vi "Load Harmonics from Test Parameter.vi"(8 "error in (no error)":errorcluster, 11 "Harmonics in":refnum<class "Harmonics.lvclass">) -> (0 "error out":errorcluster, 3 "Harmonics out":refnum<class "Harmonics.lvclass">)   [LabVIEW 2018, in "Harmonics.lvlib" / "Harmonics.lvclass"]
uses:
  Harmonics.lvclass
  C:/Sequence Automation/Plugins/Measurement Interface.lvlibp/Measurement Interface.lvclass
  Harmonics.lvclass/Harmonics.ctl
  Protected Methods/Write Harmonics.vi
  Plugins/Measurement Interface.lvlibp/Private Methods/Measurement Parameters/Read Measurement Parameters.vi
  <vilib>/Analysis/1siggen.llb/Ramp Pattern by Delta.vi
  Plugins/String Database.lvlibp/String Database.lvclass
  <vilib>/Analysis/NI_AALBase.lvlib
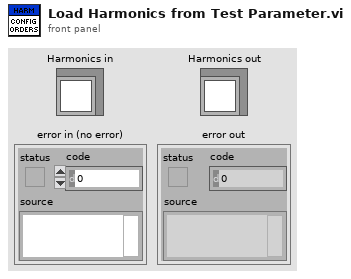
[diagram p1: front panel]
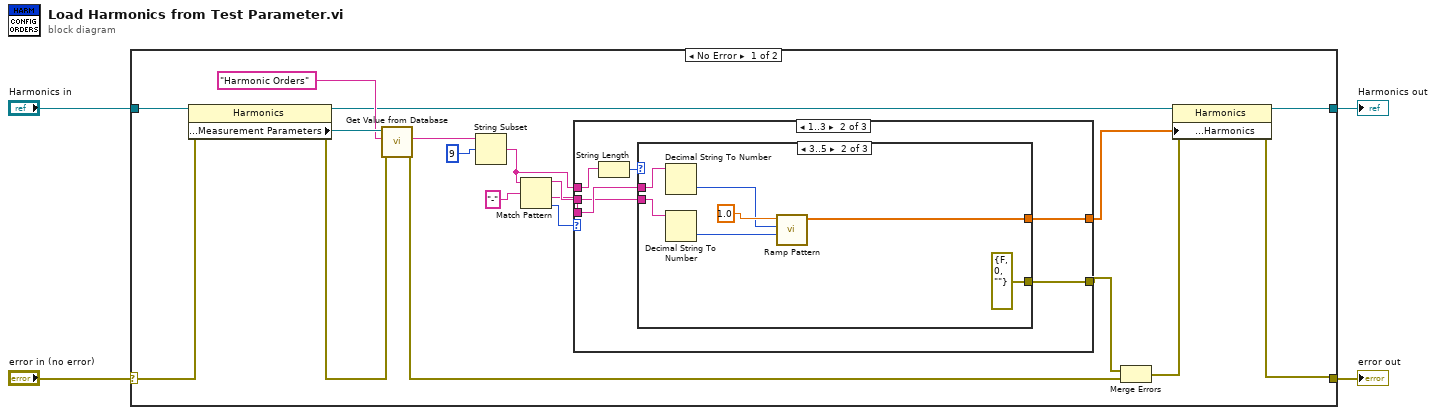
[diagram p0: block diagram]
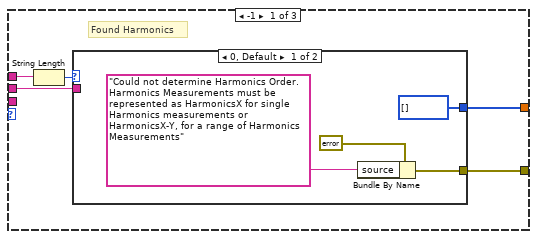
[diagram p2: hidden frame]
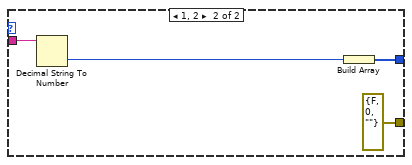
[diagram p3: hidden frame]
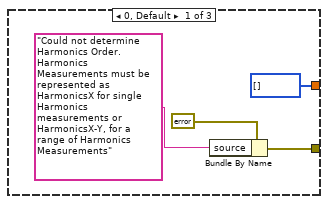
[diagram p4: hidden frame]
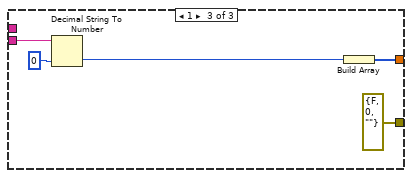
[diagram p5: hidden frame]
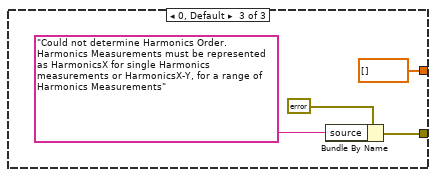
[diagram p6: hidden frame]
diagram:
  n1 = case shown="No Error" "error in (no error)" {
    selector: "error in (no error)" -> [w23 w64]
    tunnel: [w17 w64] -> w3
    tunnel: [w15 w63] -> w1
    tunnel: "Harmonics in" -> [w22 w63]
    frame No Error {
      n2 = property class="Harmonics"(reference=w22, error in=w23) -> (reference out=w16:refnum<class "Harmonics.lvclass">, error out=w20:errorcluster, "Protected Methods:Measurement Parameters"=w21:refnum<class "String Database.lvclass">)
      n3 = call "Get Value from Database.vi"("error in (no error)"=w20, "Entry Name"="Harmonic Orders", "Message in"=w21) -> ("error out"=w18:errorcluster, "Entry Value"=w7:string)  [unwired: 5 in, 2 out]
      n4 = String Subset(string=w7, offset (0)=9) -> (substring=w13:string)  [unwired: 1 in]
      n5 = Match Pattern(string=w13, regular expression="-") -> (before substring=w10:string, after substring=w9:string, offset past match=w11:i32)  [unwired: 1 in, 1 out]
      n6 = case shown="1..3" w11 {
        tunnel: [w25 w42 dbl[] [] ("Ramp Pattern")] -> w8
        tunnel: [w24 w41 w59] -> w5
        tunnel: w13 -> [w28 w37 _]
        tunnel: w10 -> [w26 w39 _]
        tunnel: w9 -> [_ w40 _]
        frame -1 {
          # "Found Harmonics"
          n7 = String Length(string=w28) -> (length=w27:i32)
          n8 = case shown="0, Default" w27 {
            tunnel: w26 -> [_ w36]
            tunnel: [i8[] [] w35] -> w25
            tunnel: [w29 errorcluster {"status"=FALSE, "code"=0, "source"=""} ("error constant")] -> w24
            frame 0, Default {
              n9 = Bundle By Name(cluster=errorcluster {"status"=TRUE, "code"=11001, "source"=""} ("error constant"), "source"="Could not determine Harmonics Order.  Harmonics Measurements must be represented as HarmonicsX for single Harmonics measurements or HarmonicsX-Y, for a range of Harmonics Measurements") -> (w29:errorcluster)
            }
            frame 1, 2 {
              n10 = Decimal String To Number(string=w36) -> (number=w33:i32)  [unwired: 2 in, 1 out]
              n11 = Build Array(w33) -> (w35:i32[])
            }
          }
        }
        frame 1..3 {
          n12 = String Length(string=w37) -> (length=w38:i32)
          n13 = case shown="3..5" w38 {
            tunnel: [i8[] [] w52 w56] -> w42
            tunnel: [w45 errorcluster {"status"=FALSE, "code"=0, "source"=""} ("error constant") errorcluster {"status"=FALSE, "code"=0, "source"=""} ("error constant")] -> w41
            tunnel: w40 -> [_ w48 _]
            tunnel: w39 -> [_ w50 w54]
            frame 0, Default {
              n14 = Bundle By Name(cluster=errorcluster {"status"=TRUE, "code"=11001, "source"=""} ("error constant"), "source"="Could not determine Harmonics Order.  Harmonics Measurements must be represented as HarmonicsX for single Harmonics measurements or HarmonicsX-Y, for a range of Harmonics Measurements") -> (w45:errorcluster)
            }
            frame 3..5 {
              n15 = Decimal String To Number(string=w48) -> (number=w47:i32)  [unwired: 2 in, 1 out]
              n16 = Decimal String To Number(string=w50) -> (number=w49:i32)  [unwired: 2 in, 1 out]
              n17 = call-poly <vilib>:"Ramp Pattern.vi"("start"=w49, "end"=w47, "delta"=1.0) -> ("Ramp Pattern"=w52:dbl[])  [unwired: 6 in, 2 out]
            }
            frame 1 {
              n18 = Decimal String To Number(string=w54, default (0L)=i8 0) -> (number=w57:i8)  [unwired: 1 in, 1 out]
              n19 = Build Array(w57) -> (w56:i8[])
            }
          }
        }
        frame 0, Default {
          n20 = Bundle By Name(cluster=errorcluster {"status"=TRUE, "code"=11001, "source"=""} ("error constant"), "source"="Could not determine Harmonics Order.  Harmonics Measurements must be represented as HarmonicsX for single Harmonics measurements or HarmonicsX-Y, for a range of Harmonics Measurements") -> (w59:errorcluster)
        }
      }
      n21 = Merge Errors(w5, w18) -> (w6:errorcluster)
      n22 = property class="Harmonics"(reference=w16, error in=w6, "Protected Methods:Harmonics"=w8) -> (reference out=w15:refnum<class "Harmonics.lvclass">, error out=w17:errorcluster)
    }
    frame Error {
    }
  }
  "error out" <- w3
  "Harmonics out" <- w1
